vi "oa_Extract XY Signal Segment (N Channels).vi"(0 "XY signals":cluster{"X":dbl[], "Y":dbl[]}[](array[cluster]) {"X" format="%.2f"; "Y" format="%.2f"}, 1 "X axis selection":u16(ring)=2 items=["Time", "Revolution", "RPM"], 2 "reset? (F)":bool, 5 "trigger indices":T1, 7 "position info in":T2, 11 "error in (no error)":errorcluster, 12 "indices end?":bool) -> (4 "XY signals out":cluster{"X":dbl[], "Y":dbl[]}[](array[cluster]) {"X" format="%.2f"; "Y" format="%.2f"}, 8 "position info out":T2, 14 "reached end?":bool, 15 "error out":errorcluster)   [LabVIEW 2017, in "SoundVib_OAUtility.lvlib"]
uses:
  <vilib>/addons/Sound and Vibration/Order Analysis/Utility/SoundVib_OAUtility.lvlib
  <vilib>/addons/Sound and Vibration/Order Analysis/Misc/OAT Position Info.ctl
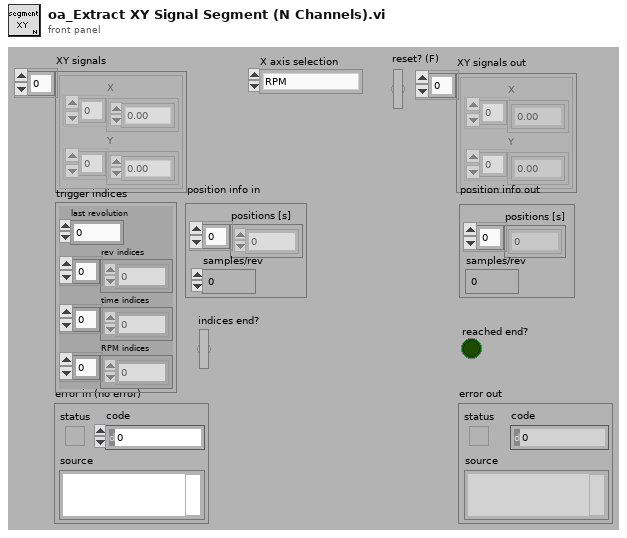
[diagram p1: front panel]
types:
  T1 = cluster{"last revolution":dbl, "rev indices":dbl[], "time indices":dbl[], "RPM indices":dbl[]}
  T2 = typedef "OAT Position Info.ctl" = cluster{"positions [s]":dbl[], "samples/rev":dbl}
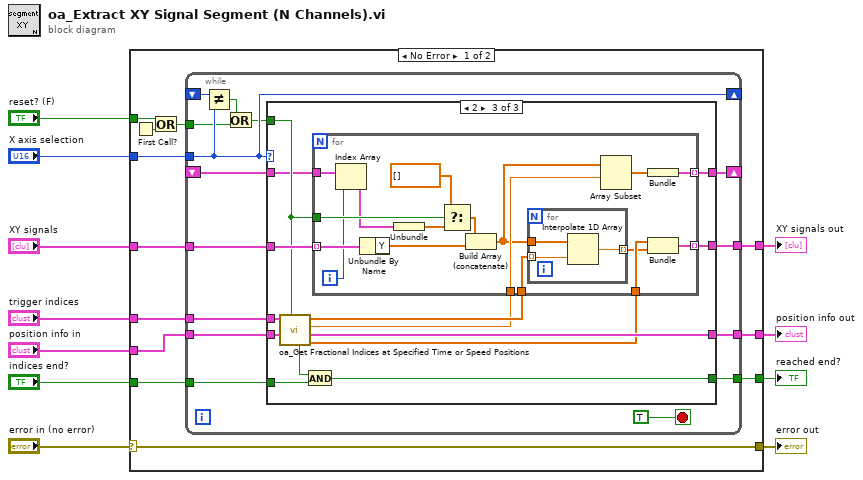
[diagram p0: block diagram]
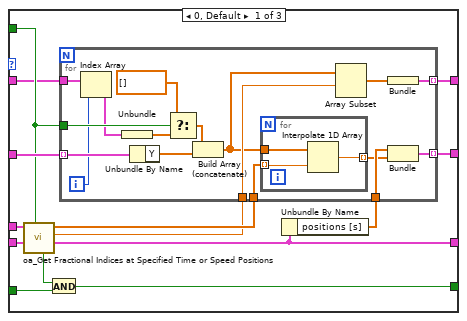
[diagram p2: hidden frame]
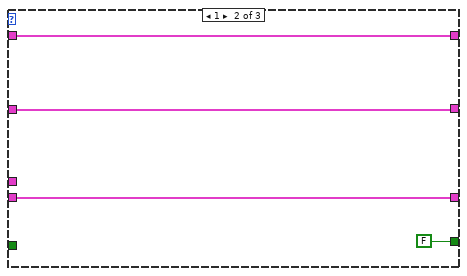
[diagram p3: hidden frame]
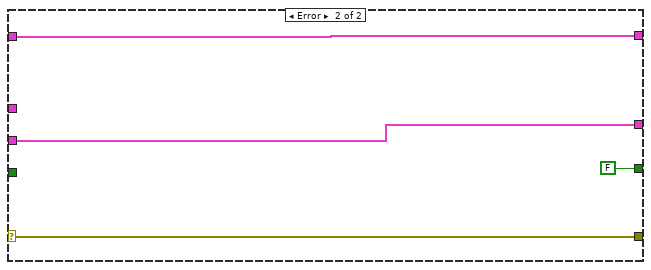
[diagram p4: hidden frame]
diagram:
  n1 = case shown="No Error" "error in (no error)" {
    selector: "error in (no error)" -> [w14 w114]
    tunnel: [w14 w114] -> w10
    tunnel: "reset? (F)" -> [w23 _]
    tunnel: "XY signals" -> [w19 w113]
    tunnel: [w20 w113] -> w7
    tunnel: "position info in" -> [w16 w112]
    tunnel: "trigger indices" -> [w17 _]
    tunnel: "X axis selection" -> [w21 _]
    tunnel: [w15 w112] -> w3
    tunnel: "indices end?" -> [w13 _]
    tunnel: [w12 FALSE] -> w1
    frame No Error {
      n2 = First Call?() -> (First Call?: T/F=w22:bool)
      n3 = Or(x=w23, y=w22) -> (x .or. y?=w18:bool)
      n4 = while {
        tunnel: w21 -> [w29]
        tunnel: [w38] -> w20
        tunnel: w19 -> [w37]
        tunnel: w18 -> [w27]
        tunnel: w17 -> [w36]
        tunnel: w16 -> [w35]
        tunnel: [w34] -> w15
        shift-right: [w32] -> _
        shift-left: _ -> [w31]
        shift-right: [w29] -> _
        shift-left: _ -> [w30]
        tunnel: w13 -> [w25]
        tunnel: [w24] -> w12
        stop <- TRUE stop-if-true
        n5 = Not Equal?(x=w30, y=w29) -> (x != y?=w26:bool)
        n6 = Or(x=w26, y=w27) -> (x .or. y?=w28:bool)
        n7 = case shown="2" w29 {
          tunnel: [w46 w76 w85] -> w38
          tunnel: w37 -> [w50 w76 w88]
          tunnel: w28 -> [w43 _ w87]
          tunnel: w36 -> [w52 _ w84]
          tunnel: w35 -> [w51 w75 w83]
          tunnel: [w48 w75 w82] -> w34
          tunnel: [w44 w74 w86] -> w32
          tunnel: w31 -> [w42 w74 w80]
          tunnel: w25 -> [w40 _ w78]
          tunnel: [w39 FALSE w77] -> w24
          frame 0, Default {
            n8 = call <vilib>:"oa_Get Fractional Indices at Specified Time or Speed Positions.vi"("reset? (F)"=w43, "position info in"=w51, "trigger indices"=w52) -> ("position info out"=w48:T2, "buffer index"=w45:dbl, "fractional indices out"=w49:dbl[], "indices buffer empty?"=w41:bool)  [unwired: 4 in, 1 out]
            n9 = And(x=w41, y=w40) -> (x .and. y?=w39:bool)
            n10 = Unbundle By Name(w48) -> ("positions [s]"=w47:dbl[])
            n11 = for {
              tunnel: w50 -> [w69] mode=indexing
              tunnel: w49 -> [w68]
              tunnel: w47 -> [w67]
              tunnel: [w66] -> w46 mode=indexing
              tunnel: w45 -> [w65]
              tunnel: [w64] -> w44 mode=indexing
              tunnel: w43 -> [w63]
              tunnel: w42 -> [w55]
              i -> [w54]
              n12 = Index Array(array=w55, index=w54) -> (element=w53:cluster{dbl[]})
              n13 = Unbundle(w53) -> (w60:dbl[])
              n14 = Unbundle By Name(w69) -> ("Y"=w58:dbl[])
              n15 = Select(t=dbl[] [], s=w63, f=w60) -> (s? t:f=w59:dbl[])
              n16 = Build Array (concatenate)(w59, w58) -> (w57:dbl[])
              n17 = for {
                tunnel: w57 -> [w72]
                tunnel: w68 -> [w71] mode=indexing
                tunnel: [w70] -> w62 mode=indexing
                n18 = Interpolate 1D Array(1:w71, 2:w72) -> (0:w70:dbl)
              }
              n19 = Array Subset(array=w57, index=w65) -> (w61:dbl[])  [unwired: 1 in]
              n20 = Bundle(w61) -> (w64:cluster{dbl[]})  [unwired: 1 in]
              n21 = Bundle("positions [s]"=w67, w62) -> (w66:cluster{"positions [s]":dbl[], dbl[]})  [unwired: 1 in]
            }
          }
          frame 1 {
          }
          frame 2 {
            n22 = call <vilib>:"oa_Get Fractional Indices at Specified Time or Speed Positions.vi"("reset? (F)"=w87, "position info in"=w83, "trigger indices"=w84) -> ("rpm indices"=w81:dbl[], "position info out"=w82:T2, "buffer index"=w89:dbl, "fractional indices out"=w90:dbl[], "indices buffer empty?"=w79:bool)  [unwired: 4 in]
            n23 = And(x=w79, y=w78) -> (x .and. y?=w77:bool)
            n24 = for {
              tunnel: w90 -> [w107]
              tunnel: w89 -> [w106]
              tunnel: w88 -> [w105] mode=indexing
              tunnel: w87 -> [w104]
              tunnel: [w103] -> w86 mode=indexing
              tunnel: [w102] -> w85 mode=indexing
              tunnel: w81 -> [w101]
              tunnel: w80 -> [w93]
              i -> [w92]
              n25 = Index Array(array=w93, index=w92) -> (element=w91:cluster{dbl[]})
              n26 = Unbundle By Name(w105) -> ("Y"=w95:dbl[])
              n27 = Unbundle(w91) -> (w98:dbl[])
              n28 = Select(t=dbl[] [], s=w104, f=w98) -> (s? t:f=w96:dbl[])
              n29 = Build Array (concatenate)(w96, w95) -> (w94:dbl[])
              n30 = for {
                tunnel: w94 -> [w110]
                tunnel: w107 -> [w109] mode=indexing
                tunnel: [w108] -> w100 mode=indexing
                n31 = Interpolate 1D Array(1:w109, 2:w110) -> (0:w108:dbl)
              }
              n32 = Array Subset(array=w94, index=w106) -> (w99:dbl[])  [unwired: 1 in]
              n33 = Bundle(w99) -> (w103:cluster{dbl[]})  [unwired: 1 in]
              n34 = Bundle("rpm indices"=w101, w100) -> (w102:cluster{"rpm indices":dbl[], dbl[]})  [unwired: 1 in]
            }
          }
        }
      }
    }
    frame Error {
    }
  }
  "error out" <- w10
  "XY signals out" <- w7
  "position info out" <- w3
  "reached end?" <- w1
